vi "Unsupported API Version Error.vi"(8 "error in (no error)":errorcluster, 10 "API version":u32, 11 "Hardware Ref in":T1 format="%.0x") -> (0 "error out":errorcluster, 3 "Hardware Ref out":T1 format="%.0x")   [LabVIEW 2017, in "Routing and Faulting Hardware API.lvlib"]
uses:
  Routing and Faulting Hardware API.lvlib
  <vilib>/NI Veristand/Custom Device API/Custom Device Item Ref.ctl
  <vilib>/NI Veristand/Custom Device API/Custom Device API.lvlib
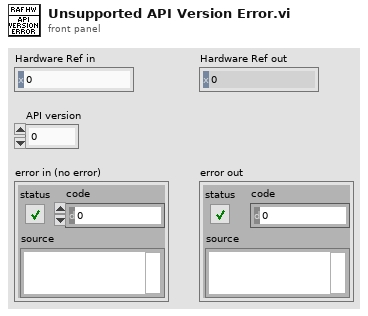
[diagram p1: front panel]
types:
  T1 = typedef "Custom Device API.lvlib/Custom Device Item Ref.ctl" = u64
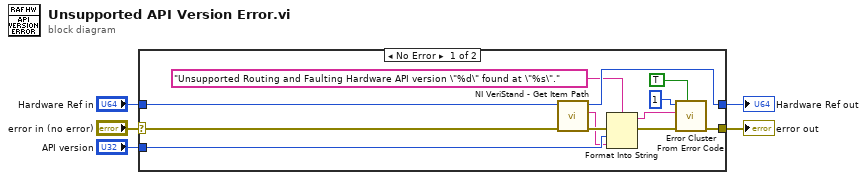
[diagram p0: block diagram]
diagram:
  n1 = case shown="No Error" "error in (no error)" {
    selector: "error in (no error)" -> [w9 w19]
    tunnel: [w17 w18] -> w5
    tunnel: "API version" -> [w16 _]
    tunnel: "Hardware Ref in" -> [w10 w18]
    tunnel: [w6 w19] -> w1
    frame No Error {
      n2 = call <vilib>:"NI VeriStand - Get Item Path.vi"("error in (no error)"=w9, "Item Ref in"=w10) -> ("error out"=w14:errorcluster, "Path"=w12:string, "Item Ref out"=w17:T1)  [unwired: 6 in, 1 out]
      n3 = Format Into String(format string="Unsupported Routing and Faulting Hardware API version \"%d\" found at \"%s\"." ("error message (\"\")"), error in=w14, w16, w12) -> (resulting string=w15:string, error out=w13:errorcluster)  [unwired: 1 in]
      n4 = call <vilib>:"Error Cluster From Error Code.vi"("show call chain? (False)"=TRUE, "error in (no error)"=w13, "error message (\"\")"=w15, "error code (0)"=1) -> ("error out"=w6:errorcluster)  [unwired: 5 in]
    }
    frame Error {
    }
  }
  "Hardware Ref out" <- w5
  "error out" <- w1
